vi "Colour Items of a JSON string control.vi"(6 "Defer Panel Updates":bool, 7 "Maximum UI Property calls":i32=-1, 8 "error in (no error)":errorcluster, 10 "String Control":refnum<vi>, 11 "JSON":string) -> (0 "error out":errorcluster)   [LabVIEW 2020, in "JSONtext.lvlib"]
doc: "Writes the input JSON to a string control and colour the elements for better readability. Note that this may be slow for large JSON structures; consider the following options\"\n1) Defer Panel Updates set to true will speed up the process by preventing display redraws untill all items are coloured. \n2) You may set a limit to number of elements that are actually coloured in order to ensure the VI completes in a reasonable amount of time (the default of -1 means no limit)."
uses:
  <vilib>/JDP Science/JSONtext/JSONtext.lvlib
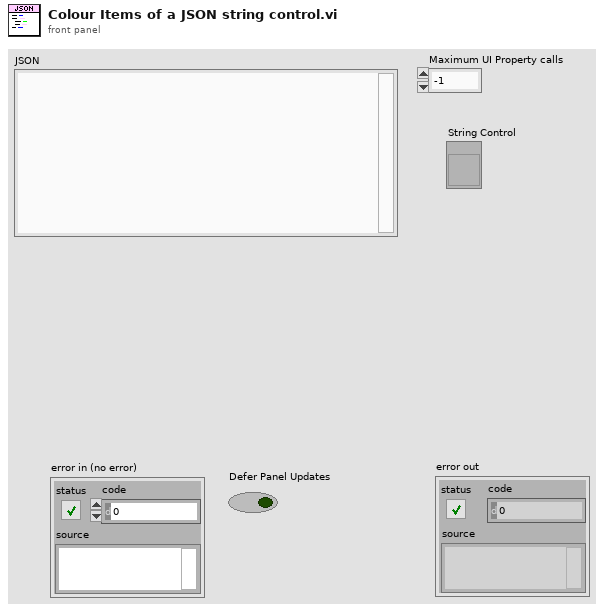
[diagram p1: front panel]
types:
  T1 = typedef "JSONtext.lvlib/Token.ctl" = cluster{"Start":i32, "End":i32, "Type":T2}
  T2 = typedef "JSONtext.lvlib/Token Type.ctl" = enum16{"Error", "Scalar", "comma", "colon", "Comment", "Down", "Up", "Line End", "Make Null", "Inline Comment", "Ignore", "junk line"}
  T3 = typedef "JSONtext.lvlib/JSON Value Type.ctl" = enum16{"Not a JSON Value", "JSON Object", "JSON Array", "String", "Number", "true", "false", "null"}
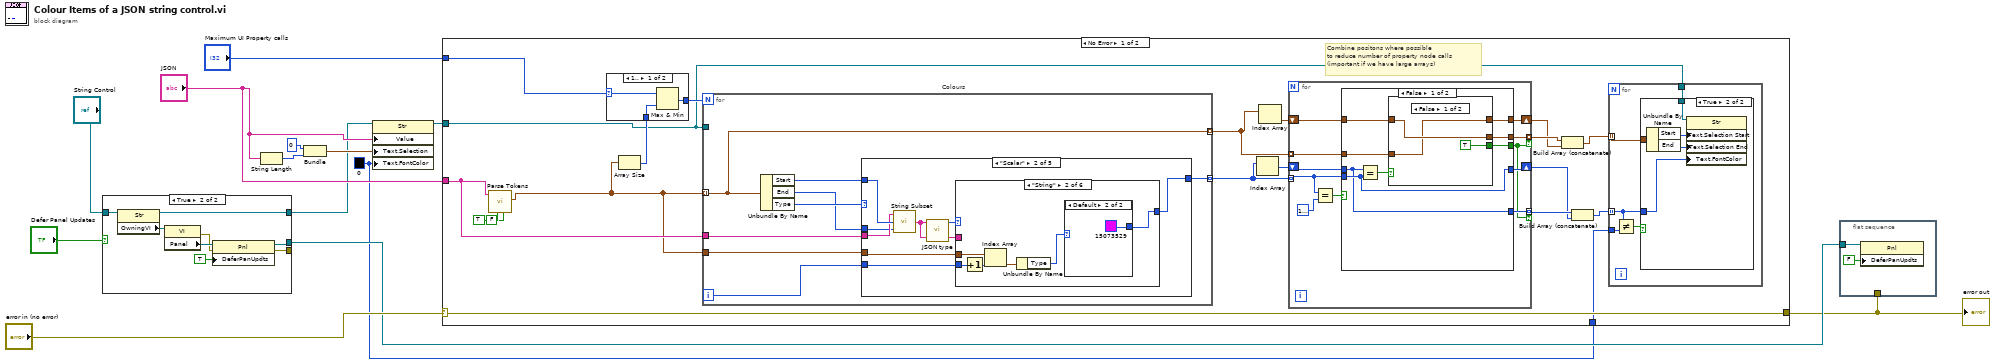
[diagram p0: block diagram]
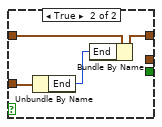
[diagram p4: hidden frame]
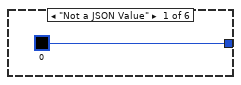
[diagram p8: hidden frame]
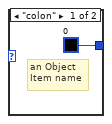
[diagram p9: hidden frame]
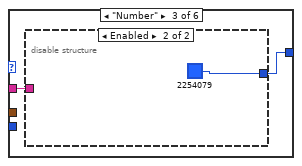
[diagram p10: hidden frame]
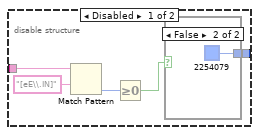
[diagram p11: hidden frame]
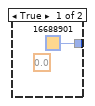
[diagram p12: hidden frame]
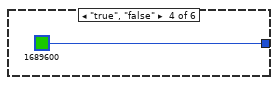
[diagram p13: hidden frame]
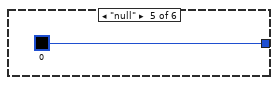
[diagram p14: hidden frame]
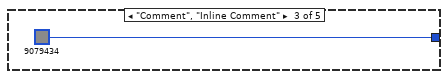
[diagram p16: hidden frame]
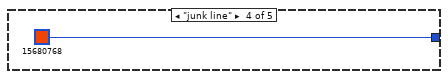
[diagram p17: hidden frame]
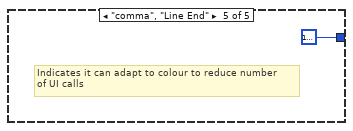
[diagram p18: hidden frame]
diagram:
  w1 = u32 0
  n1 = case shown="True" "Defer Panel Updates" {
    tunnel: "String Control" -> [w14 w22]
    tunnel: [w14 w21] -> w5
    tunnel: [_ w16] -> w3
    tunnel: [_ w15] -> _
    frame False {
    }
    frame True {
      n2 = property class="Str"(reference=w22) -> (reference out=w21:refnum<vi>, "OwningVI"=w20:refnum<vi>)  [unwired: 1 in, 1 out]
      n3 = property class="VI"(reference=w20) -> (error out=w17:errorcluster, "Panel"=w18:refnum<vi>)  [unwired: 1 in, 1 out]
      n4 = property class="Pnl"(reference=w18, error in=w17, "DeferPanUpdts"=TRUE ("Defer Panel Updates")) -> (reference out=w16:refnum<vi>, error out=w15:errorcluster)
    }
  }
  n5 = String Length(string="JSON") -> (length=w12:i32)
  n6 = Bundle("Selection Start"=u32 0, w12) -> (w11:cluster{"Selection Start":u32, i32})  [unwired: 1 in]
  n7 = property on="Property Node" class="Str"(reference=w5, "Value"="JSON", "Text.Selection"=w11, "Text.FontColor"=w1) -> (reference out=w10:refnum<vi>)  [unwired: 1 in, 1 out]
  n8 = case shown="No Error" "error in (no error)" {
    selector: "error in (no error)" -> [w39 w125]
    tunnel: w10 -> [w32 _]
    tunnel: "JSON" -> [w38 _]
    tunnel: "Maximum UI Property calls" -> [w41 _]
    tunnel: [w39 w125] -> w2
    tunnel: w1 -> [w25 _]
    frame No Error {
      # "Combine positons where possible \nto reduce number of property node calls\n(important if we have large arrays)"
      n9 = call <vilib>:"Parse Tokens.vi"("Disable LabVIEW Extensions"=FALSE, "Pretty Print"=TRUE, "JSON"=w38) -> ("Tokens"=w37:T1[])  [unwired: 8 in]
      n10 = Array Size(array=w37) -> (size(s)=w40:i32)
      n11 = case shown="1.." w41 {
        selector: w41 -> [w81 _]
        tunnel: [w83 w84] -> w42
        tunnel: w40 -> [w82 w84]
        frame 1.. {
          n12 = Max & Min(x=w81, y=w82) -> (min(x,y)=w83:i32)  [unwired: 1 out]
        }
        frame ..0 {
        }
      }
      n13 = for "Colours" {
        N: w42 -> [_]
        tunnel: w37 -> [w85] mode=indexing
        tunnel: w32 -> [_]
        tunnel: w38 -> [w91]
        tunnel: w37 -> [w88]
        tunnel: [w86] -> w34 mode=indexing
        tunnel: [w85] -> w35 mode=indexing
        i -> [w87]
        n14 = Unbundle By Name(w85) -> ("Start"=w90:i32, "End"=w89:i32, "Type"=w92:T2)
        n15 = case shown="\"Scalar\"" w92 {
          tunnel: [_ w100 u32 9079434 u32 15680768 u32 16777216] -> w86
          tunnel: w91 -> [_ w98 _ _ _]
          tunnel: w90 -> [_ w99 _ _ _]
          tunnel: w89 -> [_ w97 _ _ _]
          tunnel: w88 -> [_ w95 _ _ _]
          tunnel: w87 -> [_ w94 _ _ _]
          frame Default {
          }
          frame "Scalar" {
            n16 = call <vilib>:"String Subset.vi"("Offset past End"=w97, "Start offset"=w99, "JSON"=w98) -> ("substring"=w93:string)  [unwired: 2 in]
            n17 = call <vilib>:"JSON type.vi"("JSON"=w93) -> ("JSON Value Type"=w96:T3)  [unwired: 9 in, 1 out]
            n18 = case shown="\"String\"" w96 {
              tunnel: [u32 0 w107 w111 u32 1689600 u32 0 _] -> w100
              tunnel: w95 -> [_ w106 _ _ _ _]
              tunnel: w94 -> [_ w104 _ _ _ _]
              tunnel: w93 -> [_ _ w110 _ _ _]
              frame "Not a JSON Value" {
              }
              frame "String" {
                n19 = Increment(x=w104) -> (x+1=w105:i32)
                n20 = Index Array(array=w106, index=w105) -> (element=w103:T1)
                n21 = Unbundle By Name(w103) -> ("Type"=w102:T2)
                n22 = case shown="Default" w102 {
                  tunnel: [u32 0 u32 15073529] -> w107
                  frame "colon" {
                    # "an Object\nItem name"
                  }
                  frame Default {
                  }
                }
              }
              frame "Number" {
                n23 = disable-structure shown="Enabled" {
                  disable-tunnel: [w116 u32 2254079] -> w111
                  disable-tunnel: w110 -> [w113 _]
                  frame Disabled {
                    n24 = Match Pattern(string=w113, regular expression="[eE\\.IN]") -> (offset past match=w114:i32)  [unwired: 1 in, 3 out]
                    n25 = Greater Or Equal To 0?(x=w114) -> (x >= 0?=w112:bool)
                    n26 = case shown="False" w112 {
                      tunnel: [u32 16688901 u32 2254079] -> w116
                      frame True {
                        (unwired) 0.0
                      }
                      frame False {
                      }
                    }
                  }
                  frame Enabled {
                  }
                }
              }
              frame "true", "false" {
              }
              frame "null" {
              }
              frame Default {
              }
            }
          }
          frame "Comment", "Inline Comment" {
          }
          frame "junk line" {
          }
          frame "comma", "Line End" {
            # "Indicates it can adapt to colour to reduce number\nof UI calls"
          }
        }
      }
      n27 = Index Array(array=w34) -> (element=w33:u32)  [unwired: 1 in]
      n28 = Index Array(array=w35) -> (element=w36:T1)  [unwired: 1 in]
      n29 = for {
        shift-right: [w60] -> w29
        shift-left: w36 -> [w61]
        tunnel: w35 -> [w59] mode=indexing
        tunnel: w34 -> [w58] mode=indexing
        shift-right: [w55] -> w27
        shift-left: w33 -> [w63]
        tunnel: [w62] -> w31 mode=indexing if=w53
        tunnel: [w54] -> w28 mode=indexing if=w53
        n30 = Equal?(x=w58, y=u32 16777216) -> (x = y?=w56:bool)
        n31 = case shown="False" w56 {
          tunnel: w63 -> [w64 w79]
          tunnel: [w70 _] -> w62
          tunnel: w61 -> [w69 w80]
          tunnel: [w68 _] -> w53
          tunnel: [w67 w80] -> w60
          tunnel: w59 -> [w66 _]
          tunnel: w58 -> [w65 _]
          tunnel: [w65 w79] -> w55
          tunnel: [w64 _] -> w54
          frame False {
            n32 = Equal?(x=w64, y=w65) -> (x = y?=w71:bool)
            n33 = case shown="False" w71 {
              tunnel: [w74 _] -> w70
              tunnel: w69 -> [w74 w78]
              tunnel: [TRUE _] -> w68
              tunnel: [w72 w77] -> w67
              tunnel: w66 -> [w72 w76]
              frame False {
              }
              frame True {
                n34 = Unbundle By Name(w76) -> ("End"=w75:i32)
                n35 = Bundle By Name(cluster=w78, "End"=w75) -> (w77:T1)
              }
            }
          }
          frame True {
            # "Comma --> allow it to take\non same colour as both sides\n(in order to reduce number of\nUI calls)"
          }
        }
      }
      n36 = Build Array (concatenate)(w31, w29) -> (w30:T1[])
      n37 = Build Array (concatenate)(w28, w27) -> (w26:u32[])
      n38 = for {
        tunnel: w32 -> [w47]
        tunnel: w30 -> [w46] mode=indexing
        tunnel: w26 -> [w45] mode=indexing
        tunnel: w25 -> [w44]
        n39 = Not Equal?(x=w45, y=w44) -> (x != y?=w43:bool)
        n40 = case shown="True" w43 {
          tunnel: w47 -> [_ w52]
          tunnel: w46 -> [_ w51]
          tunnel: w45 -> [_ w48]
          frame False {
          }
          frame True {
            n41 = Unbundle By Name(w51) -> ("Start"=w50:i32, "End"=w49:i32)
            n42 = property on="Property Node" class="Str"(reference=w52, "Text.Selection Start"=w50, "Text.Selection End"=w49, "Text.FontColor"=w48) -> ()  [unwired: 1 in, 2 out]
          }
        }
      }
    }
    frame Error {
    }
  }
  "error out" <- w2
  n43 = flat-sequence {
    tunnel: w3 -> [w126]
    tunnel: w2 -> [_]
    frame #0 {
      n44 = property class="Pnl"(reference=w126, "DeferPanUpdts"=FALSE ("Defer Panel Updates")) -> ()  [unwired: 1 in, 2 out]
    }
  }
